vi "group Sync Read Tx Rx Packet.vi"(11 "group_num":i32) -> ()   [LabVIEW 2021, in "dxl_x86_c.lvlib"]
doc: "WINDECLSPEC void groupSyncReadTxRxPacket (int group_num);"
uses:
  dxl_x86_c.lvlib
  dxl_x86_c.dll
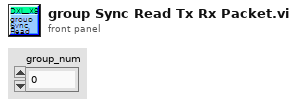
[diagram p1: front panel]
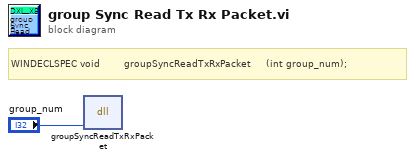
[diagram p0: block diagram]
diagram:
  # "WINDECLSPEC void        groupSyncReadTxRxPacket     (int group_num);"
  n1 = dll-call lib="C:/Users/ashek/Desktop/ashekim/ws/DynamixelSDK/labview/labview/dxl_x86_c.*" fn="groupSyncReadTxRxPacket"("group_num"="group_num") -> ()  [unwired: 5 in, 2 out]
